vi "Calculate IMOrder given F1, F2, Fim.vi"(9 "IM Frequency":dbl, 10 "F2 (Carrier 2)":dbl, 11 "F1 (Carrier 1)":dbl) -> (0 "Low-Side?":bool, 1 "IM Order String":string, 2 "IM Order":u8, 3 "BaseImOrder":i32)   [LabVIEW 2011]
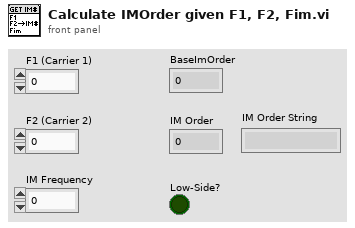
[diagram p1: front panel]
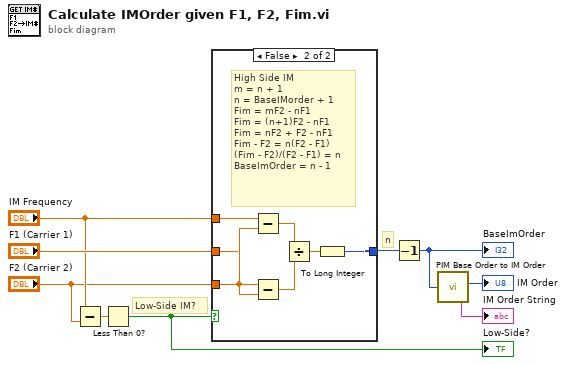
[diagram p0: block diagram]
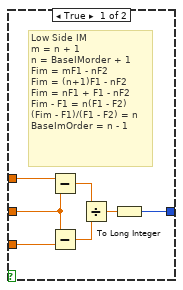
[diagram p2: hidden frame]
diagram:
  # "Low-Side IM?"
  # "n"
  n1 = Subtract(x="IM Frequency", y="F2 (Carrier 2)") -> (x-y=w5:dbl)
  n2 = Less Than 0?(x=w5) -> (x < 0?=w2:bool)
  "Low-Side?" <- w2
  n3 = case shown="False" w2 {
    tunnel: "IM Frequency" -> [w16 w23]
    tunnel: "F1 (Carrier 1)" -> [w15 w17]
    tunnel: "F2 (Carrier 2)" -> [w14 w18]
    tunnel: [w10 w19] -> w8
    frame True {
      # "Low Side IM\nm = n + 1\nn = BaseIMorder + 1\nFim = mF1 - nF2\nFim = (n+1)F1 - nF2\nFim = nF1 + F1 - nF2\nFim - F1 = n(F1 - F2)\n(Fim - F1)/(F1 - F2) = n\nBaseImOrder = n - 1"
      n4 = Subtract(x=w16, y=w15) -> (x-y=w12:dbl)
      n5 = Subtract(x=w15, y=w14) -> (x-y=w13:dbl)
      n6 = Divide(x=w12, y=w13) -> (x/y=w11:dbl)
      n7 = To Long Integer(number=w11) -> (32bit integer=w10:i32)
    }
    frame False {
      # "High Side IM\nm = n + 1\nn = BaseIMorder + 1\nFim = mF2 - nF1\nFim = (n+1)F2 - nF1\nFim = nF2 + F2 - nF1\nFim - F2 = n(F2 - F1)\n(Fim - F2)/(F2 - F1) = n\nBaseImOrder = n - 1"
      n8 = Subtract(x=w23, y=w18) -> (x-y=w21:dbl)
      n9 = Subtract(x=w18, y=w17) -> (x-y=w22:dbl)
      n10 = Divide(x=w21, y=w22) -> (x/y=w20:dbl)
      n11 = To Long Integer(number=w20) -> (32bit integer=w19:i32)
    }
  }
  n12 = Decrement(x=w8) -> (x-1=w4:i32)
  "BaseImOrder" <- w4
  n13 = call "PIM Base Order to IM Order.vi"("Base Order (0)"=w4) -> ("IM Order"=→"IM Order":u8, "IM Order String"=→"IM Order String":string)  [unwired: 4 in]
